vi "mkShowSettingsDialog.vi"(10 "IMAQ Refnum":refnum<k11>, 11 "Camera (in)":T1={"Gain [1-4]"=100.0, "Offset"=100, "Mode"=0, "ROIs"=[], "ROI Size"={"X"=0, "Y"=0}, "Number of buffers"=40, "Use hardware multiple-ROI?"=TRUE, "GenericCameraConfig"={"Framerate (Hz)"=60, "Exposure time (us)"=5000, "Image size"={"Width"=1280, "Height"=1024}, "Number of buffers"=30}} {"Mode" min=50}) -> (3 "Camera (out)":T1={"Gain [1-4]"=100.0, "Offset"=100, "Mode"=0, "ROIs"=[], "ROI Size"={"X"=0, "Y"=0}, "Number of buffers"=40, "Use hardware multiple-ROI?"=TRUE, "GenericCameraConfig"={"Framerate (Hz)"=60, "Exposure time (us)"=5000, "Image size"={"Width"=1280, "Height"=1024}, "Number of buffers"=30}} {"Mode" min=50})   [LabVIEW 2011]
uses:
  CameraConfig.ctl
  Main/Camera/GenericCameraConfigType.ctl
panel:
  in  "Serial send":bool
  out "Serial response:":string
  in  "Serial cmd:":string
  in  "Get":bool
  in  "Reset camera":bool
  in  "Set":bool
  in  "Number of ROIs to compute\nmax framerate for:":i32=2
  out "Max exposure time":i32
  out "Maximum framerate (press apply first)":i32
  in  "Revert":bool
  in  "Camera":T1={"Gain [1-4]"=100.0, "Offset"=2, "Mode"=75, "ROIs"=[], "ROI Size"={"X"=120, "Y"=120}, "Number of buffers"=40, "Use hardware multiple-ROI?"=FALSE, "GenericCameraConfig"={"Framerate (Hz)"=60, "Exposure time (us)"=5000, "Image size"={"Width"=1280, "Height"=1024}, "Number of buffers"=30}} {"Mode" min=50}
  in  "OK":bool
  in  "Apply":bool
  # "us"
  # "us"
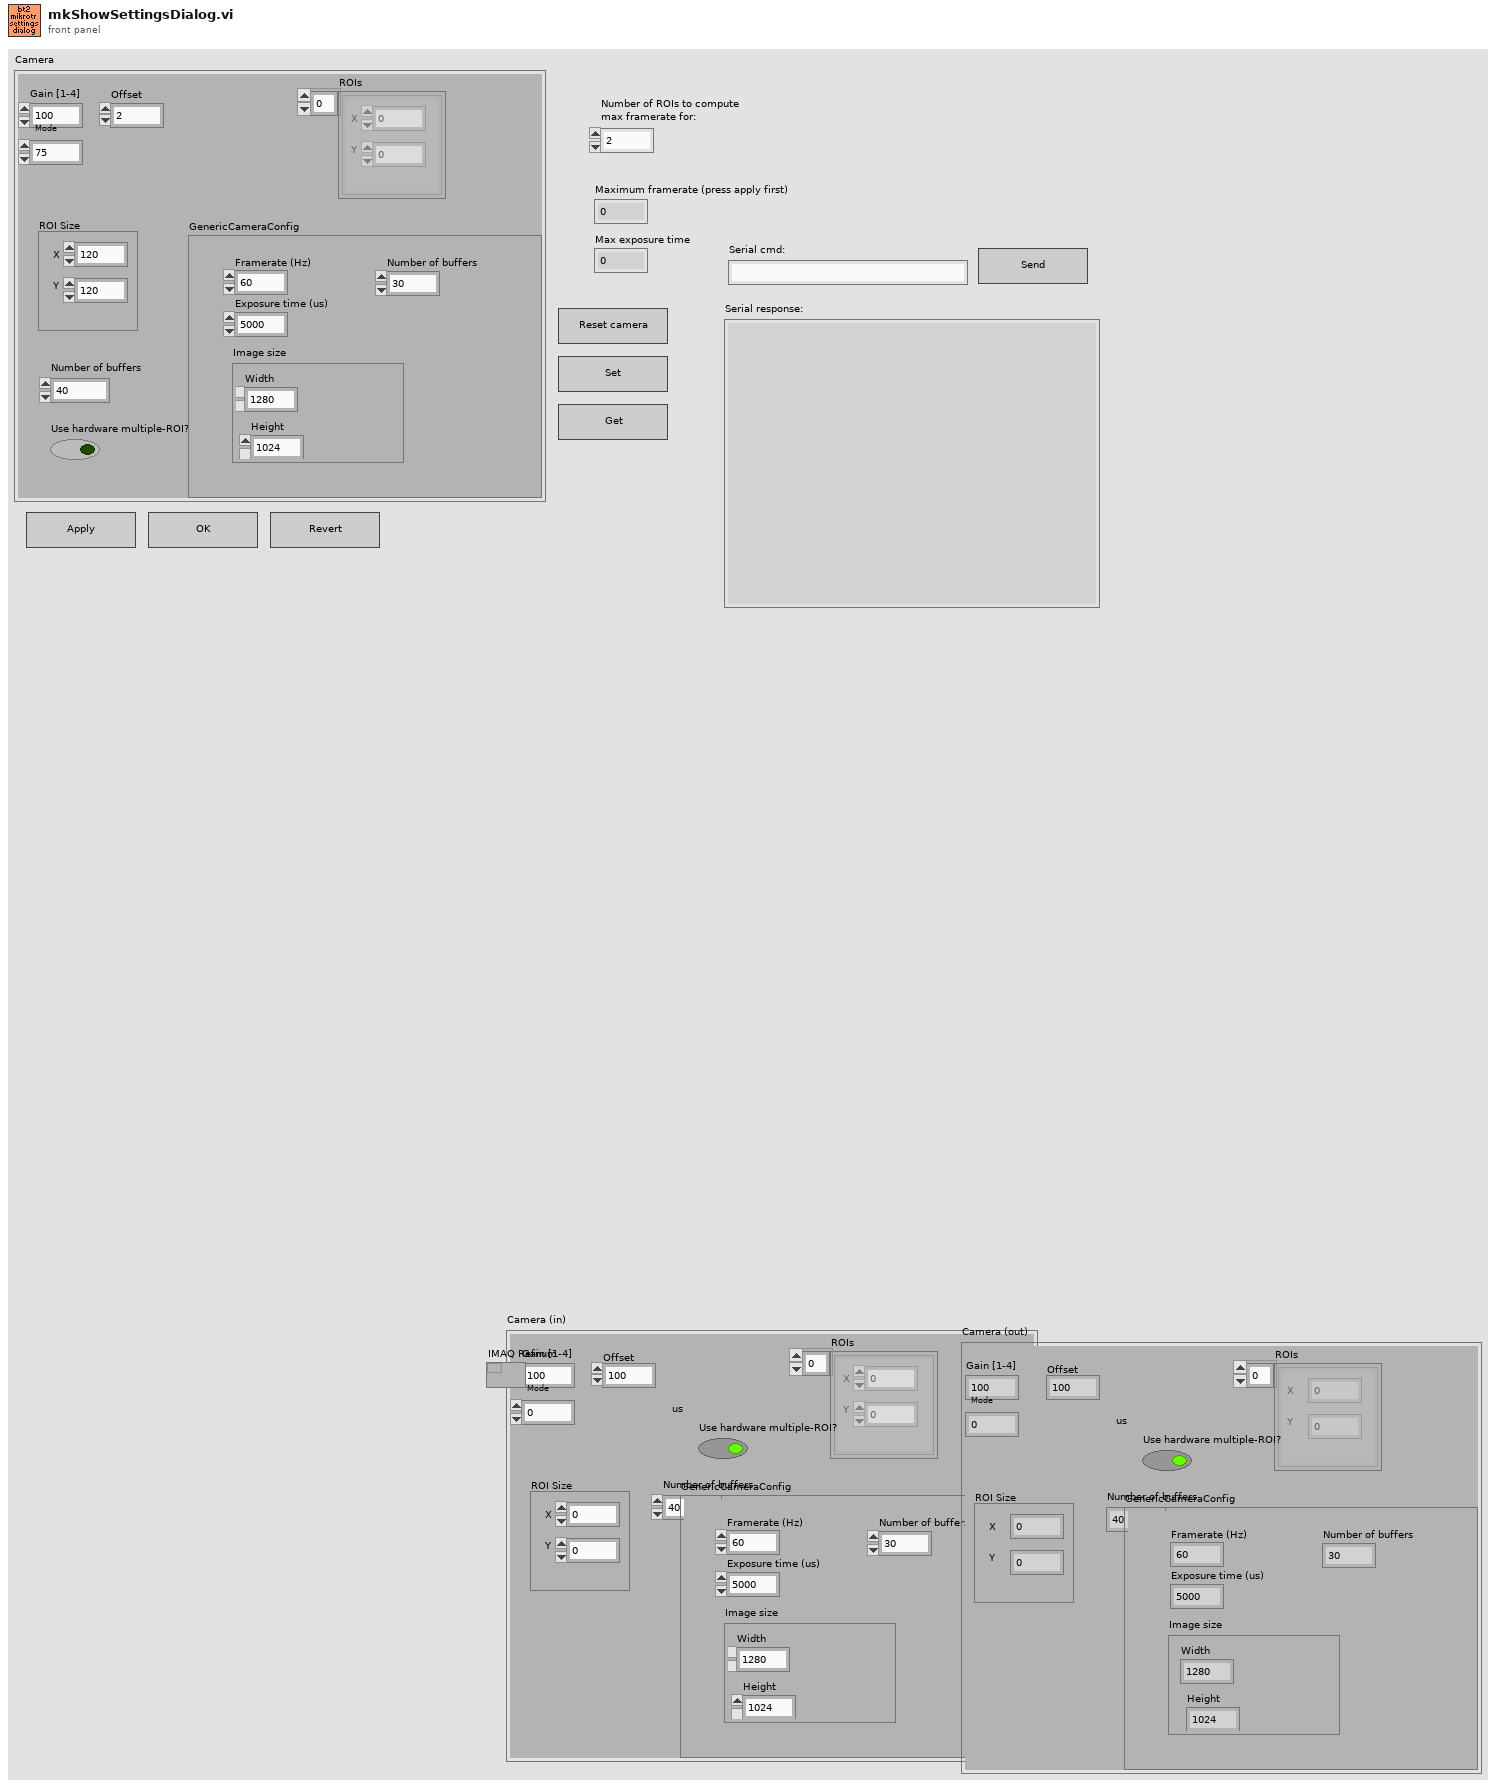
[diagram p1: front panel]
types:
  T1 = typedef "CameraConfig.ctl" = cluster{"Gain [1-4]":sgl, "Offset":i16, "Mode":i16, "ROIs":cluster{"X":i32, "Y":i32}[], "ROI Size":cluster{"X":i32, "Y":i32}, "Number of buffers":i32, "Use hardware multiple-ROI?":bool, "GenericCameraConfig":T2}
  T2 = typedef "GenericCameraConfigType.ctl" = cluster{"Framerate (Hz)":i32, "Exposure time (us)":i32, "Image size":cluster{"Width":i32, "Height":i32}, "Number of buffers":i32}
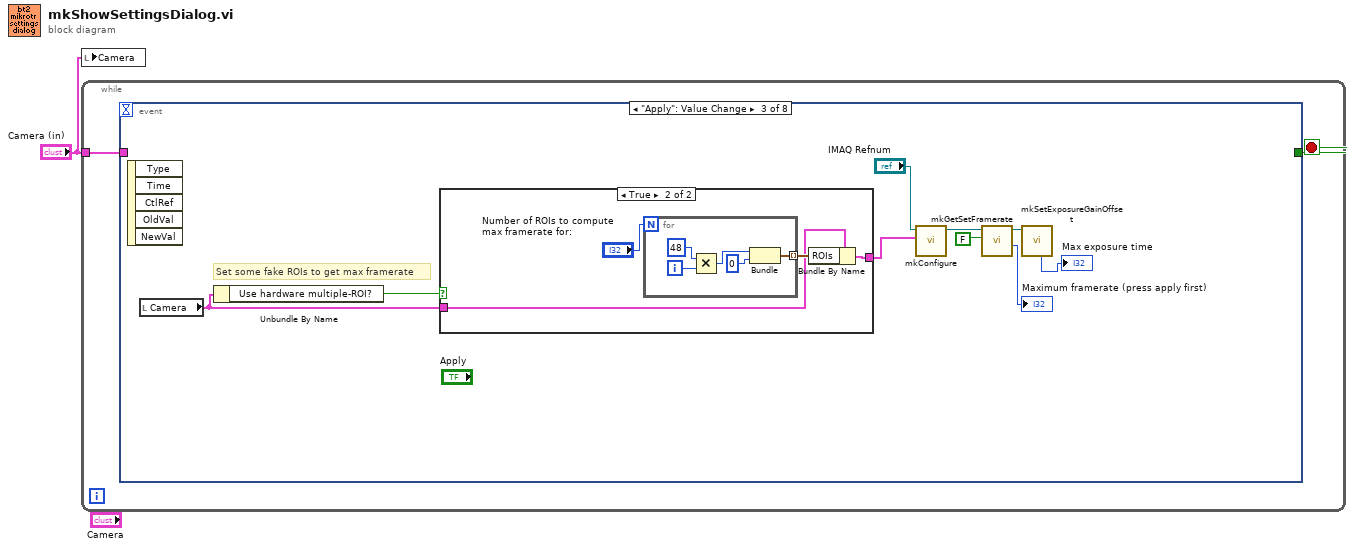
[diagram p0: block diagram]
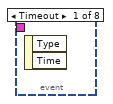
[diagram p2: hidden frame]
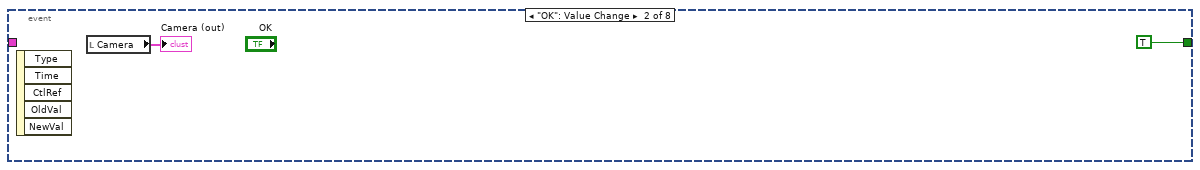
[diagram p3: hidden frame]
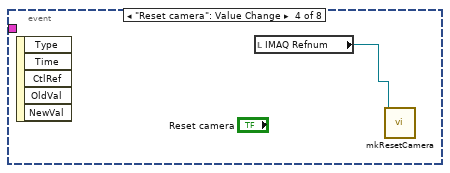
[diagram p5: hidden frame]
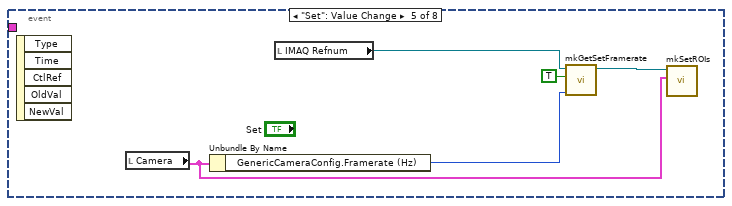
[diagram p6: hidden frame]
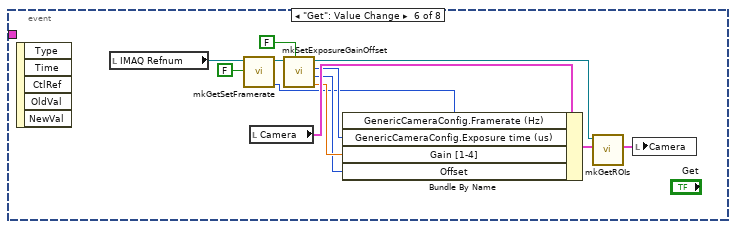
[diagram p7: hidden frame]
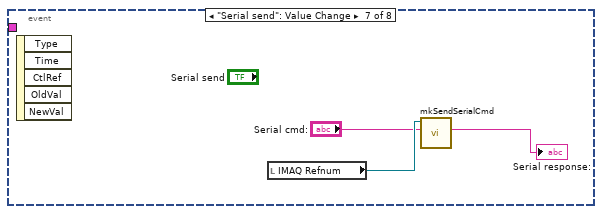
[diagram p8: hidden frame]
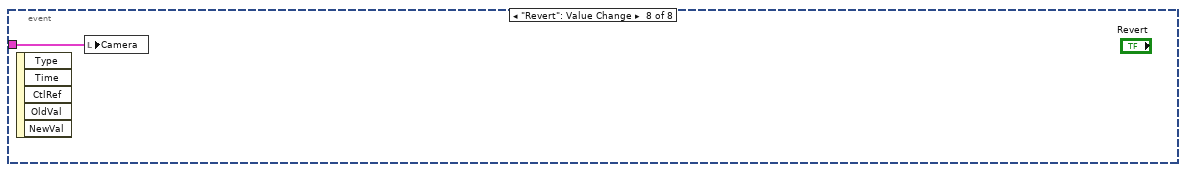
[diagram p9: hidden frame]
diagram:
  n1 = local write "Camera"("Camera (in)") -> ()
  n2 = while {
    tunnel: "Camera (in)" -> [w2]
    stop <- w3 stop-if-true
    n3 = event shown="[2] \"Apply\": Value Change" {
      selector: _ -> [_ _ _ _ _ _ _ _]
      dyn-events: _ -> [_ _ _ _ _ _ _ _]
      timeout: _ -> [_ _ _ _ _ _ _ _]
      tunnel: [_ TRUE _ _ _ _ _ _] -> w3
      tunnel: w2 -> [_ _ _ _ _ _ _ w46]
      event Timeout {
        n4 = event-data() -> ()  [unwired: 1 in, 2 out]
      }
      event "OK": Value Change {
        n5 = event-data() -> ()  [unwired: 1 in, 5 out]
        n6 = local read "Camera"() -> (→"Camera (out)":T1)
      }
      event "Apply": Value Change {
        # "Set some fake ROIs to get max framerate"
        n7 = event-data() -> ()  [unwired: 1 in, 5 out]
        n8 = local read "Camera"() -> (w11:T1)
        n9 = Unbundle By Name(w11) -> ("Use hardware multiple-ROI?"=w12:bool)
        n10 = case shown="True" w12 {
          tunnel: w11 -> [w15 w17]
          tunnel: [w15 w16] -> w13
          frame False {
          }
          frame True {
            n11 = for {
              N: "Number of ROIs to compute\nmax framerate for:" -> [_]
              tunnel: [w20] -> w18 mode=indexing
              i -> [w23]
              n12 = Multiply(x=48, y=w23) -> (x*y=w21:i32)
              n13 = Bundle(w21, 0) -> (w20:cluster{i32, i32})  [unwired: 1 in]
            }
            n14 = Bundle By Name(cluster=w17, "ROIs"=w18) -> (w16:T1)
          }
        }
        n15 = call "mkConfigure.vi"("Camera in"=w13, "IMAQ Session"="IMAQ Refnum") -> ("IMAQ Refnum out"=w10:refnum<k11>)  [unwired: 8 in, 1 out]
        n16 = call "mkGetSetFramerate.vi"("Set? (F)"=FALSE, "IMAQ Refnum out"=w10) -> ("Maximum framerate"=→"Maximum framerate (press apply first)":i32, "IMAQ Refnum (out)"=w7:refnum<k11>)  [unwired: 6 in, 2 out]
        n17 = call "mkSetExposureGainOffset.vi"("IMAQ Refnum in"=w7) -> ("Max exposure time"=→"Max exposure time":i32)  [unwired: 5 in, 5 out]
      }
      event "Reset camera": Value Change {
        n18 = event-data() -> ()  [unwired: 1 in, 5 out]
        n19 = local read "IMAQ Refnum"() -> (w25:refnum<k11>)
        n20 = call "mkResetCamera.vi"("IMAQ Refnum in"=w25) -> ()  [unwired: 10 in, 1 out]
      }
      event "Set": Value Change {
        n21 = event-data() -> ()  [unwired: 1 in, 5 out]
        n22 = local read "Camera"() -> (w26:T1)
        n23 = Unbundle By Name(w26) -> ("GenericCameraConfig.Framerate (Hz)"=w28:i32)
        n24 = local read "IMAQ Refnum"() -> (w30:refnum<k11>)
        n25 = call "mkGetSetFramerate.vi"("Framerate"=w28, "Set? (F)"=TRUE, "IMAQ Refnum out"=w30) -> ("IMAQ Refnum (out)"=w27:refnum<k11>)  [unwired: 5 in, 3 out]
        n26 = call "mkSetROIs.vi"("Camera in"=w26, "IMAQ Refnum in"=w27) -> ()  [unwired: 9 in, 1 out]
      }
      event "Get": Value Change {
        n27 = event-data() -> ()  [unwired: 1 in, 5 out]
        n28 = local read "IMAQ Refnum"() -> (w42:refnum<k11>)
        n29 = call "mkGetSetFramerate.vi"("Set? (F)"=FALSE, "IMAQ Refnum out"=w42) -> ("Framerate"=w33:i32, "IMAQ Refnum (out)"=w39:refnum<k11>)  [unwired: 6 in, 2 out]
        n30 = local read "Camera"() -> (w37:T1)
        n31 = call "mkSetExposureGainOffset.vi"("Set? (F)"=FALSE, "IMAQ Refnum in"=w39) -> ("Gain"=w36:dbl, "Offset"=w35:u32, "Exposure time"=w34:i32, "IMAQ Refnum out"=w38:refnum<k11>)  [unwired: 4 in, 2 out]
        n32 = Bundle By Name(cluster=w37, "GenericCameraConfig.Framerate (Hz)"=w33, "GenericCameraConfig.Exposure time (us)"=w34, "Gain [1-4]"=w36, "Offset"=w35) -> (w32:T1)
        n33 = call "mkGetROIs.vi"("Camera settings"=w32, "IMAQ Refnum in"=w38) -> ("Camera settings (out)"=w31:T1)  [unwired: 8 in, 1 out]
        n34 = local write "Camera"(w31) -> ()
      }
      event "Serial send": Value Change {
        n35 = event-data() -> ()  [unwired: 1 in, 5 out]
        n36 = local read "IMAQ Refnum"() -> (w45:refnum<k11>)
        n37 = call "mkSendSerialCmd.vi"("String"="Serial cmd:", "IMAQ Refnum in"=w45) -> ("String Read"=→"Serial response:":string)  [unwired: 6 in, 3 out]
      }
      event "Revert": Value Change {
        n38 = event-data() -> ()  [unwired: 1 in, 5 out]
        n39 = local write "Camera"(w46) -> ()
      }
    }
  }
